vi "My_Server_v1.vi"   [LabVIEW 2019]
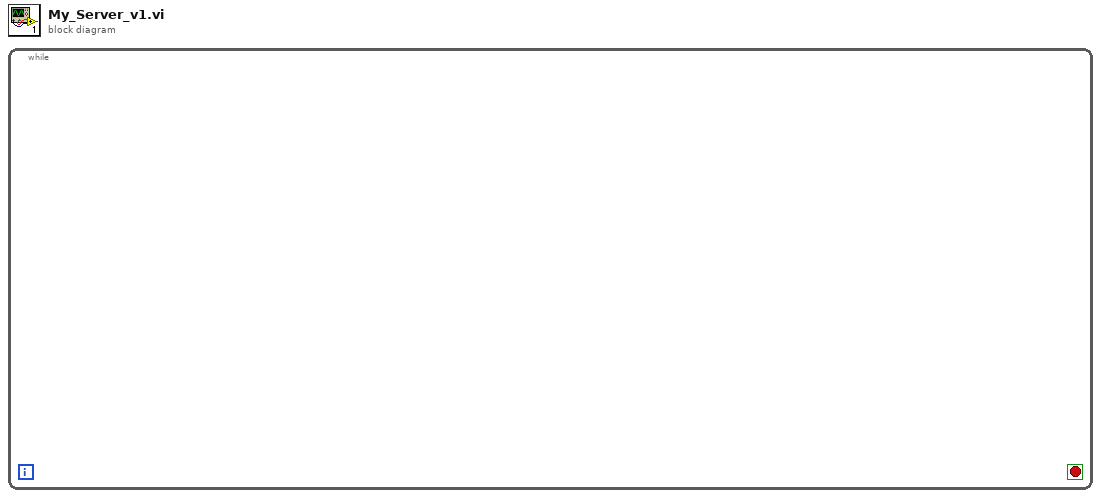
[diagram p0: block diagram]
diagram:
  n1 = while {
    stop <- _ stop-if-true
  }
